vi "niRFUtil CFG INI File.vi"(0 "File In":path, 5 "Buffer Size (1024 bytes)":i32=1024, 11 "error in (no error)":errorcluster, 13 "Action (Read)":enum16{"Read", "Write", "Delete"}(ring)) -> (4 "dup File":path, 6 "Sections":string[](array[string]), 15 "error out":errorcluster)   [LabVIEW 2015, in "niRFUtil.lvlib"]
doc: "This VI allows the user to read or write entries in a text file that is in the standard Windows INI file format. \n\nThe Read action returns an array of strings of all of the section names in the INI file.\n\nThe Write action creates an empty file if the file doesn't already exist, and will not do anything if the file already exists.\n\nThe Delete action will delete the INI file.\n\n(c) Copyright 2007, National Instruments, Inc. This software may not be duplicated, sold, or distributed without written consent from National Instruments."
uses:
  niRFUtil.lvlib
  kernel32.dll
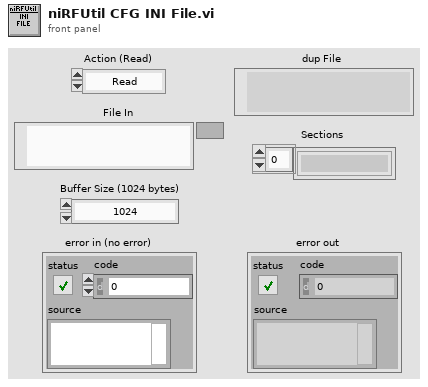
[diagram p1: front panel]
types:
  T1 = enum16{"open", "replace", "create", "open or create", "replace or create", "replace or create with confirmation"}
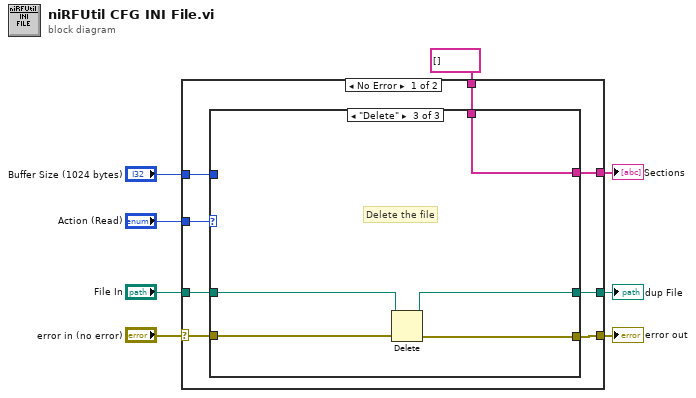
[diagram p0: block diagram]
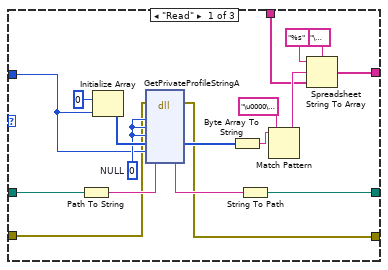
[diagram p2: hidden frame]
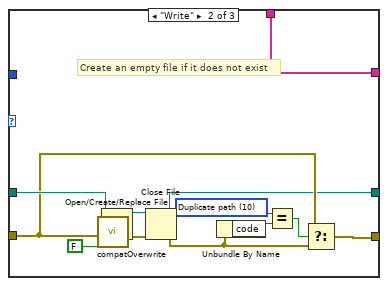
[diagram p3: hidden frame]
diagram:
  n1 = case shown="No Error" "error in (no error)" {
    selector: "error in (no error)" -> [w11 w54]
    tunnel: [w14 w54] -> w8
    tunnel: [w16 w55] -> w5
    tunnel: "Action (Read)" -> [w15 _]
    tunnel: "File In" -> [w10 w53]
    tunnel: string[] [] -> [w13 w55]
    tunnel: "Buffer Size (1024 bytes)" -> [w12 _]
    tunnel: [w9 w53] -> w1
    frame No Error {
      n2 = case shown="\"Delete\"" w15 {
        tunnel: [w25 w44 w49] -> w16
        tunnel: w11 -> [w19 w40 w51]
        tunnel: w10 -> [w31 w46 w50]
        tunnel: [w18 w42 w52] -> w14
        tunnel: w13 -> [w24 w44 w49]
        tunnel: w12 -> [w20 _ _]
        tunnel: [w17 w35 w48] -> w9
        frame "Read" {
          w21 = 0  # NULL
          n3 = Path To String(path=w31) -> (string=w30:string)
          n4 = Initialize Array(u8 0, w20) -> (w23:u8[])
          n5 = dll-call lib="Kernel32.dll" fn="GetPrivateProfileStringA" label="Read"(error in=w19, "AppName"=w21, "KeyName"=w21, "Default"=w21, "ReturnedString"=w23, "Size"=w20, "FileName"=w30) -> (error out=w18:errorcluster, "ReturnedString"=w34:u8[], "FileName"=w29:string)  [unwired: 6 in, 2 out]
          n6 = Byte Array To String(unsigned byte array=w34) -> (string=w33:string)
          n7 = String To Path(string=w29) -> (path=w17:path)
          n8 = Match Pattern(string=w33, regular expression="\u0000\u0000") -> (before substring=w26:string)  [unwired: 4 out]
          n9 = Spreadsheet String To Array(delimiter (Tab)="\u0000", format string="%s", spreadsheet string=w26, array type (2D Dbl)=w24) -> (array=w25:string[])
        }
        frame "Write" {
          w38 = u16 10 items=["No error", "Argument error", "Memory is full", "Out of zone", "End of file", "File already open", "Generic file I/O error", "File not found", "File permission error", "Disk is full", "Duplicate path", "Too many files open", "System feature not enabled", "Resource file not found", "Cannot add resource", "Resource not found", "Image not found", "Image memory error", "Pen does not exist", "Config type invalid", "Config token not found", "Config parse error", "Config memory error", "Bad external code format", "Bad external code offset", "External code not present", "Null window", "Destroy window error", "Null menu", "Print aborted", "Bad print record", "Print driver error", "Windows error during printing", "Memory error during printing", "Print dialog error", "Generic print error", "Invalid device refnum", "Device not found", "Device parameter error", "Device unit error", "Cannot open device", "Device call aborted", "Generic error", "Cancelled by user", "Object ID too low", "Object ID too high", "Object not in heap", "Unknown heap", "Unknown object (invalid DefProc)", "Unknown object (DefProc not in table)", "Message out of range", "Invalid (null) method", "Unknown message", "Manager call not supported", "Bad address", "Network operation in progress", "Network operation timed out", "Connection is busy", "Network attribute not supported", "Network error", "Address in use", "System out of memory", "Connection aborted", "Connection refused", "Not connected", "Already connected", "Connection closed", "Initialization error (interapplication manager)", "Bad occurrence", "Wait on unbound occurrence handler", "Occurrence queue overflow", "Datalog type conflict", "Unused", "Unrecognized type (interapplication manager)", "Memory corrupt", "Failed to make temporary DLL", "Old CIN version", "Drag socket not found", "Failed to load drop-object", "Failed to register OLE object", "Failed to release OLE object", "Format specifier type mismatch", "Unknown format specifier", "Too few format specifiers", "Too many format specifiers", "Scan failed", "Newer CIN version", "OLE Convert", "Runtime menu error", "Password tampered", "Unknown error code"]
          # "Create an empty file if it does not exist"
          n10 = call <vilib>:"compatOverwrite.vi"("overwrite (F)"=FALSE) -> ("overwrite?"=w36:T1)
          n11 = Open/Create/Replace File(file path (use dialog)=w46, error in=w40, operation (0:open)=w36) -> (refnum out=w47:refnum<file>, error out=w43:errorcluster)  [unwired: 4 out]
          n12 = Close File(refnum=w47, error in=w43) -> (path=w35:path, error out=w41:errorcluster)
          n13 = Unbundle By Name(w41) -> ("code"=w39:i32)
          n14 = Equal?(x=w38, y=w39) -> (x = y?=w37:bool)
          n15 = Select(t=w40, s=w37, f=w41) -> (s? t:f=w42:errorcluster)
        }
        frame "Delete" {
          # "Delete the file"
          n16 = Delete(path (use dialog)=w50, error in=w51) -> (deleted path=w48:path, error out=w52:errorcluster)  [unwired: 4 out]
        }
      }
    }
    frame Error {
    }
  }
  "error out" <- w8
  "Sections" <- w5
  "dup File" <- w1
